vi "build sequence.vi"(1 "Enum":enum16{"logarithmic", "linear"}(ring), 2 "amount":u32, 3 "min":u32, 4 "max":u32) -> (0 "Array - Numeric":i32[](array[numeric]))   [LabVIEW 2021]
uses:
  68a9031c-5d2d-4209-a6c2-63c16a2c4737.vi
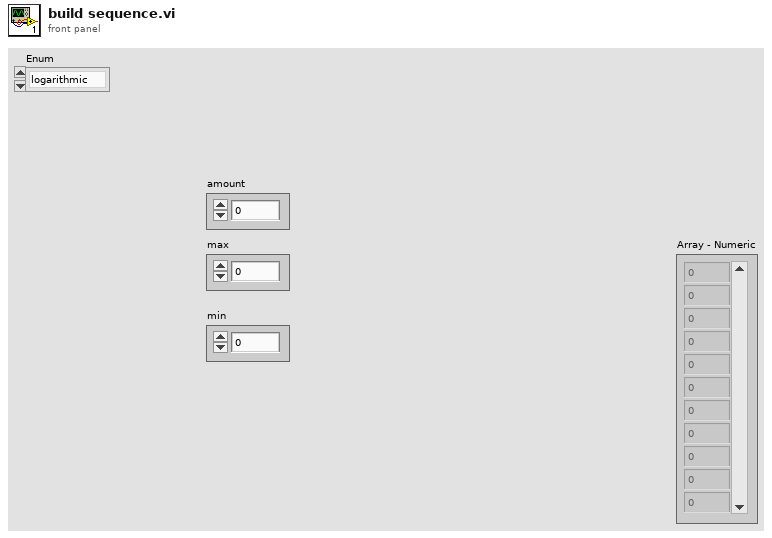
[diagram p1: front panel]
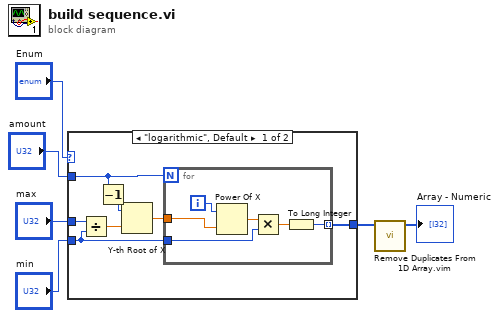
[diagram p0: block diagram]
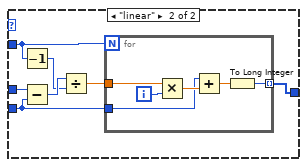
[diagram p2: hidden frame]
diagram:
  n1 = case shown="\"logarithmic\", Default" "Enum" {
    tunnel: "amount" -> [w8 w26]
    tunnel: "max" -> [w11 w23]
    tunnel: [w12 w24] -> w3
    tunnel: "min" -> [w9 w21]
    frame "logarithmic", Default {
      n2 = Divide(x=w11, y=w9) -> (x/y=w10:dbl)
      n3 = Decrement(x=w8) -> (x-1=w7:u32)
      n4 = Y-th Root of X(1:w10, 2:w7) -> (0:w13:dbl)
      n5 = for {
        N: w8 -> [_]
        tunnel: w13 -> [w19]
        tunnel: [w17] -> w12 mode=indexing
        tunnel: w9 -> [w14]
        i -> [w18]
        n6 = Power Of X(1:w19, 2:w18) -> (0:w15:dbl)
        n7 = Multiply(x=w15, y=w14) -> (x*y=w16:dbl)
        n8 = To Long Integer(number=w16) -> (32bit integer=w17:i32)
      }
    }
    frame "linear" {
      n9 = Decrement(x=w26) -> (x-1=w20:u32)
      n10 = Subtract(x=w23, y=w21) -> (x-y=w22:u32)
      n11 = Divide(x=w22, y=w20) -> (x/y=w25:dbl)
      n12 = for {
        N: w26 -> [_]
        tunnel: w25 -> [w32]
        tunnel: [w31] -> w24 mode=indexing
        tunnel: w21 -> [w28]
        i -> [w27]
        n13 = Multiply(x=w32, y=w27) -> (x*y=w30:dbl)
        n14 = Add(x=w28, y=w30) -> (x+y=w29:dbl)
        n15 = To Long Integer(number=w29) -> (32bit integer=w31:i32)
      }
    }
  }
  n16 = call "Remove Duplicates From 1D Array.vim"("array"=w3) -> ("array with duplicates removed"=→"Array - Numeric":i32[])  [unwired: 10 in]
